vi "Set Cell Value Excel.vi"(4 "background color (w)":u32=16776960 format="%06x", 6 "outside border":T1={"on/off"=FALSE, "weight"=2, "color"=0} {"weight" items=["xlHairline"=1, "xlMedium"=-4138, "xlThick"=4, "xlThin"=2]}, 7 "font":T2={"font name"="", "font size"=10.0, "bold"=1, "italic"=0, "underline"=0, "strike through"=0, "font color"=16777216} {"font size" format="%0.2f"; "strike through" items=["Strk Unchanged", "Strk Yes", "Strk No"]; "underline" items=["Und Unchanged", "Und Yes", "Und No"]; "italic" items=["Ital Unchanged", "Ital Yes", "Ital No"]; "bold" items=["Bold Unchanged", "Bold Yes", "Bold No"]}, 8 "error in (no error)":errorcluster, 9 "end (-1, -1)":cluster{"row":i32, "column":i32}, 10 "Data":dbl, 11 "NI_report in":refnum<class "NI_report.lvclass">) -> (0 "error out":errorcluster, 3 "NI_report out":refnum<class "NI_report.lvclass">)   [LabVIEW 2023]
uses:
  <vilib>/Utility/NIReport.llb/NI_report.lvclass
  <vilib>/addons/_office/_exclsub.llb/font.ctl
  <vilib>/addons/_office/NI_ReportGenerationToolkit.lvlib
  <vilib>/Utility/NIReport.llb/Excel/NI_Excel.lvclass
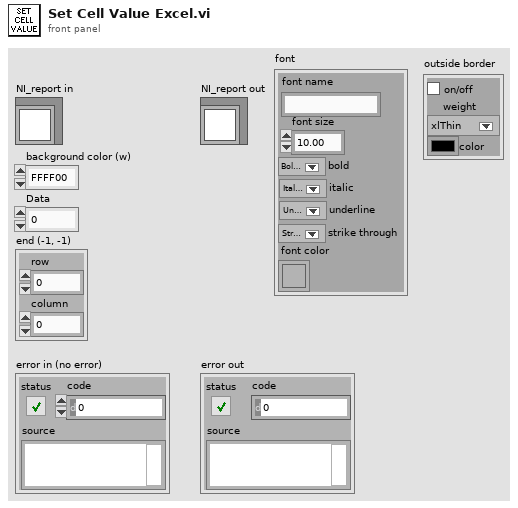
[diagram p1: front panel]
types:
  T1 = cluster{"on/off":bool, "weight":i32, "color":u32}
  T2 = typedef "NI_ReportGenerationToolkit.lvlib/font.ctl" = cluster{"font name":string, "font size":dbl, "bold":u16, "italic":u16, "underline":u16, "strike through":u16, "font color":u32}
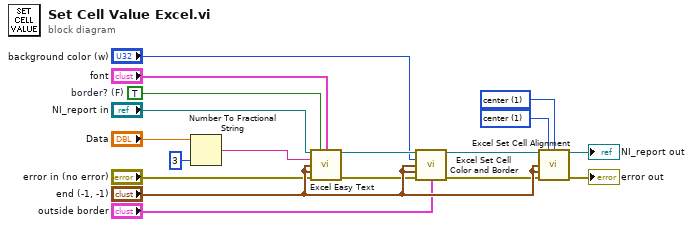
[diagram p0: block diagram]
diagram:
  w4 = TRUE  # border? (F)
  w16 = 1 items=["left", "center", "right"] ("horizontal alignment (left)")
  w15 = 1 items=["top", "center", "bottom"] ("vertical alignment (top)")
  n1 = Number To Fractional String(number="Data", precision (6)=i16 3) -> (F-format string=w7:string)  [unwired: 2 in]
  n2 = call <vilib>:"Excel Easy Text.vi"("report in"="NI_report in", "border? (F)"=w4, "font"="font", "text"=w7, "start (-1, -1)"="end (-1, -1)", "end (-1, -1)"="end (-1, -1)", "error in (no error)"="error in (no error)") -> ("report out"=w10:refnum<class "NI_report.lvclass">, "error out"=w11:errorcluster)  [unwired: 4 in, 3 out]
  n3 = call <vilib>:"Excel Set Cell Color and Border.vi"("report in"=w10, "outside border"="outside border", "background color (w)"="background color (w)", "start (-1, -1)"="end (-1, -1)", "end (-1, -1)"="end (-1, -1)", "error in (no error)"=w11) -> ("report out"=w12:refnum<class "NI_report.lvclass">, "error out"=w13:errorcluster)  [unwired: 8 in]
  n4 = call <vilib>:"Excel Set Cell Alignment.vi"("report in"=w12, "vertical alignment (top)"=w15, "horizontal alignment (left)"=w16, "start (-1, -1)"="end (-1, -1)", "end (-1, -1)"="end (-1, -1)", "error in (no error)"=w13) -> ("report out"=→"NI_report out":refnum<class "NI_report.lvclass">, "error out"=→"error out":errorcluster)  [unwired: 8 in]
